vi "Validate_Destination_For_Amalgamation.vi"(10 "Destination":refnum<class "AB_Destination.lvclass">, 11 "AB_Source.lvclass":refnum<class "AB_Source.lvclass">) -> (3 "Valid?":bool)   [LabVIEW 2020, in "AB_Source.lvclass"]
uses:
  <vilib>/AppBuilder/AB_Classes/Source/AB_Source.lvclass
  <vilib>/AppBuilder/AB_Classes/Destination/AB_Destination.lvclass
  <vilib>/AppBuilder/AB_Classes/Source/AB_Source.lvclass/AB_Source.ctl
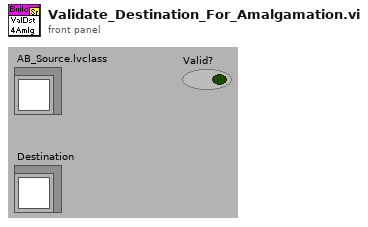
[diagram p1: front panel]
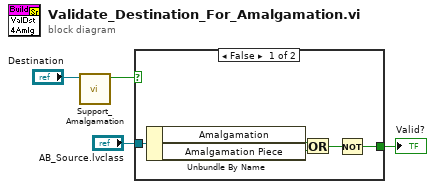
[diagram p0: block diagram]
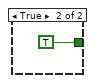
[diagram p2: hidden frame]
diagram:
  n1 = call-dynamic "Support_Amalgamation.vi"("AB_Destination in"="Destination") -> ("Supports amalgamations?"=w1:bool)  [unwired: 1 in, 9 out]
  n2 = case shown="False" w1 {
    tunnel: [w5 TRUE] -> w4
    tunnel: "AB_Source.lvclass" -> [w7 _]
    frame False {
      n3 = Unbundle By Name(w7) -> ("Amalgamation"=w8:bool, "Amalgamation Piece"=w9:bool)
      n4 = Or(x=w8, y=w9) -> (x .or. y?=w6:bool)
      n5 = Not(x=w6) -> (.not. x?=w5:bool)
    }
    frame True {
    }
  }
  "Valid?" <- w4
